vi "Set Timeouts.vi"(8 "error in":errorcluster, 9 "write operation timeout":i32=5000, 10 "read operation timeout":i32=5000, 11 "Modbus master in":refnum<class "Modbus Master.lvclass">) -> (0 "error out":errorcluster, 3 "Modbus master out":refnum<class "Modbus Master.lvclass">)   [LabVIEW 2014, in "MyLib.lvlib" / "Modbus Master.lvclass"]
doc: "Provides a simple function for defining the timeout of read and write operations on the bus. This function takes effect immediately, and will change the timeouts of any future operations using the instance returned by <B>Modbus master out</B>. Multiple timeout settings can be used simultaneously by forking the wire."
uses:
  Modbus Master.lvclass
  Modbus API.lvclass/Modbus API.ctl
  Transmission Data Unit/Transmission Data Unit.lvclass/Transmission Data Unit.ctl
  Modbus API.lvclass
  Transmission Data Unit/Transmission Data Unit.lvclass
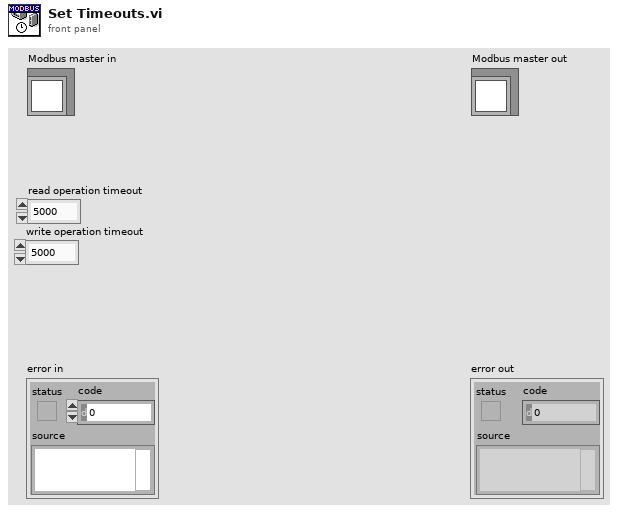
[diagram p1: front panel]
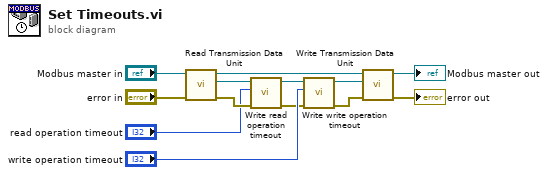
[diagram p0: block diagram]
diagram:
  n1 = call "Read Transmission Data Unit.vi"("error in"="error in", "Modbus instance in"="Modbus master in") -> ("error out"=w11:errorcluster, "transmission data unit"=w12:refnum<class "Transmission Data Unit.lvclass">, "Modbus instance out"=w13:refnum<class "Modbus Master.lvclass">)  [unwired: 7 in]
  n2 = call "Write read operation timeout.vi"("error in (no error)"=w11, "read operation timeout"="read operation timeout", "transmission data unit in"=w12) -> ("error out"=w6:errorcluster, "transmission data unit out"=w9:refnum<class "Transmission Data Unit.lvclass">)  [unwired: 7 in]
  n3 = call "Write write operation timeout.vi"("error in (no error)"=w6, "write operation timeout"="write operation timeout", "transmission data unit in"=w9) -> ("error out"=w5:errorcluster, "transmission data unit out"=w10:refnum<class "Transmission Data Unit.lvclass">)  [unwired: 7 in]
  n4 = call "Write Transmission Data Unit.vi"("error in"=w5, "transmission data unit"=w10, "Modbus instance in"=w13) -> ("error out"=→"error out":errorcluster, "Modbus instance out"=→"Modbus master out":refnum<class "Modbus Master.lvclass">)  [unwired: 7 in]
